vi "Stop Core.vi"(10 "final error code":i32, 11 "Test Node View in":refnum<class "Test Node View.lvclass">) -> (3 "Test Node View out":refnum<class "Test Node View.lvclass">)   [LabVIEW 2013, in "Test Node View.lvlib" / "Test Node View.lvclass"]
doc: "(<B>Filename</B>: Actor Framework.lvlib:Actor.lvclass:Stop Core.vi)\n\nDefines what the actor does before it stops. Use the <B>final error code</B> input to determine whether the actor shut down in response to an error.\n\nBy default, this method does nothing. A descendant class may override it to define behavior, such as shutting down any processes the actor initiated in its override of the Actor Core method."
uses:
  Test Node View.lvclass
  <vilib>/ActorFrameworkMVC/View Actor/View Actor.lvclass
  Test Node View.lvclass/Test Node View.ctl
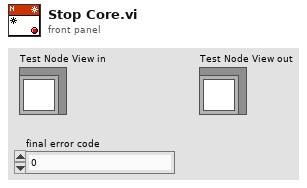
[diagram p1: front panel]
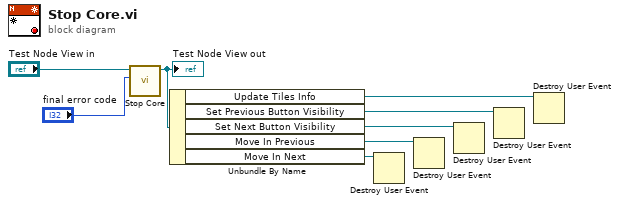
[diagram p0: block diagram]
diagram:
  n1 = call-parent "Stop Core.vi"("final error code"="final error code", "Actor in"="Test Node View in") -> ("Actor out"=w6:refnum<class "Test Node View.lvclass">)  [unwired: 9 in]
  "Test Node View out" <- w6
  n2 = Unbundle By Name(w6) -> ("Update Tiles Info"=w5:refnum<user-event>, "Set Previous Button Visibility"=w3:refnum<user-event>, "Set Next Button Visibility"=w4:refnum<user-event>, "Move In Previous"=w2:refnum<user-event>, "Move In Next"=w1:refnum<user-event>)
  n3 = Destroy User Event(user event=w1) -> ()  [unwired: 1 in, 1 out]
  n4 = Destroy User Event(user event=w2) -> ()  [unwired: 1 in, 1 out]
  n5 = Destroy User Event(user event=w4) -> ()  [unwired: 1 in, 1 out]
  n6 = Destroy User Event(user event=w3) -> ()  [unwired: 1 in, 1 out]
  n7 = Destroy User Event(user event=w5) -> ()  [unwired: 1 in, 1 out]
